vi "Preset Filenames.vi"(5 "FileNameInput References":T1, 7 "Filename Flag Cluster":T2, 10 "LIN TXT Datei Name":string, 11 "EPA TXT Datei Name":string) -> ()   [LabVIEW 2020, in "Linearisierung v2.lvlib"]
uses:
  Linearisierung V2/Linearisierung v2.lvlib
panel:
  out "Fehler (Ausgang)":errorcluster
  in  "Fehler (Eingang, kein Fehler)":errorcluster
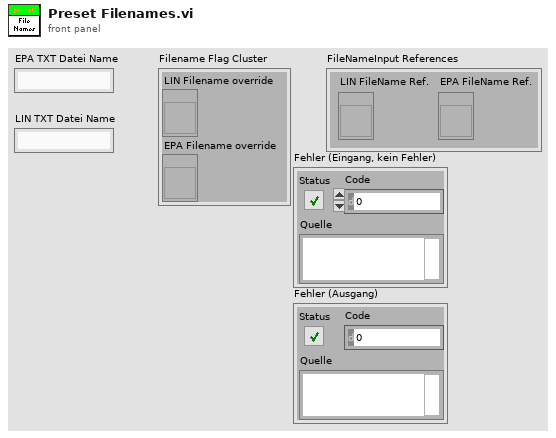
[diagram p1: front panel]
types:
  T1 = cluster{"LIN FileName Ref.":refnum<vi>, "EPA FileName Ref.":refnum<vi>}
  T2 = cluster{"LIN Filename override":refnum<vi>, "EPA Filename override":refnum<vi>}
  T3 = typedef "Checkbox(boolsch).ctl" = bool
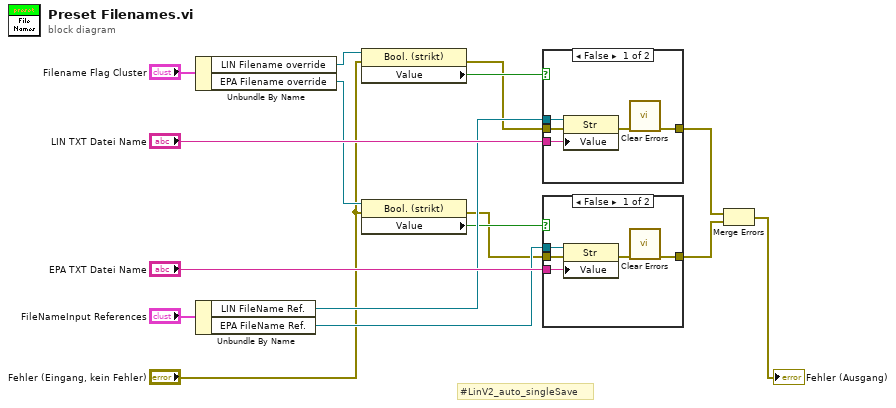
[diagram p0: block diagram]
diagram:
  # "#LinV2_auto_singleSave"
  n1 = Unbundle By Name("Filename Flag Cluster") -> ("LIN Filename override"=w10:refnum<vi>, "EPA Filename override"=w9:refnum<vi>)
  n2 = Unbundle By Name("FileNameInput References") -> ("LIN FileName Ref."=w12:refnum<vi>, "EPA FileName Ref."=w11:refnum<vi>)
  n3 = property class="Bool. (strikt)"(reference=w10, error in="Fehler (Eingang, kein Fehler)") -> (error out=w5:errorcluster, "Value"=w8:T3)  [unwired: 1 out]
  n4 = property class="Bool. (strikt)"(reference=w9, error in="Fehler (Eingang, kein Fehler)") -> (error out=w4:errorcluster, "Value"=w7:T3)  [unwired: 1 out]
  n5 = case shown="False" w8 {
    tunnel: "LIN TXT Datei Name" -> [w21 _]
    tunnel: w12 -> [w20 _]
    tunnel: w5 -> [w19 w22]
    tunnel: [w17 w22] -> w3
    frame False {
      n6 = property class="Str"(reference=w20, error in=w19, "Value"=w21) -> (error out=w18:errorcluster)  [unwired: 1 out]
      n7 = call <vilib>:"Clear Errors.vi"("error in (no error)"=w18) -> ("error out"=w17:errorcluster)  [unwired: 5 in, 1 out]
    }
    frame True {
    }
  }
  n8 = case shown="False" w7 {
    tunnel: "EPA TXT Datei Name" -> [w27 _]
    tunnel: w11 -> [w26 _]
    tunnel: w4 -> [w25 w28]
    tunnel: [w23 w28] -> w2
    frame False {
      n9 = property class="Str"(reference=w26, error in=w25, "Value"=w27) -> (error out=w24:errorcluster)  [unwired: 1 out]
      n10 = call <vilib>:"Clear Errors.vi"("error in (no error)"=w24) -> ("error out"=w23:errorcluster)  [unwired: 5 in, 1 out]
    }
    frame True {
    }
  }
  n11 = Merge Errors(w3, w2) -> (→"Fehler (Ausgang)":errorcluster)
